vi "UI.vi"(8 "error in (no error)":errorcluster, 11 "Node Ptr":T1 format="%.0x") -> (0 "error out":errorcluster)   [LabVIEW 2017, in "Modules.lvlib" / "9210.lvclass"]
uses:
  9210.lvclass
  <vilib>/NI Veristand/Custom Device API/Custom Device Item Ref.ctl
  RSI Module/SubPanel Command.ctl
  C:/Users/nitest/Documents/NI/niveristand-scan-engine-module-libraries/Source/RSI Module/RSI Module.lvclass
  9210.lvclass/9210.ctl
  RSI Module/RSI Module.lvclass
  <vilib>/NI Veristand/Custom Device API/Custom Device API.lvlib
panel:
  in  "Units":u8(ring) caption="Measurement Units" items=["Raw Volts", "Degrees Kelvin", "Degrees Celsius", "Degrees Fahrenheit", "Degrees Rankine"]
  in  "Type":u8(ring) caption="Thermocouple Type" items=["J", "K", "T", "E", "R", "S", "N", "B"]
  in  "Channels":i32[](listbox)=[0]
  in  "SubPanel Event":refnum<user-event>
  in  "Header":cluster{"Section Name":string}={"Section Name"="NI 9210 Settings"}
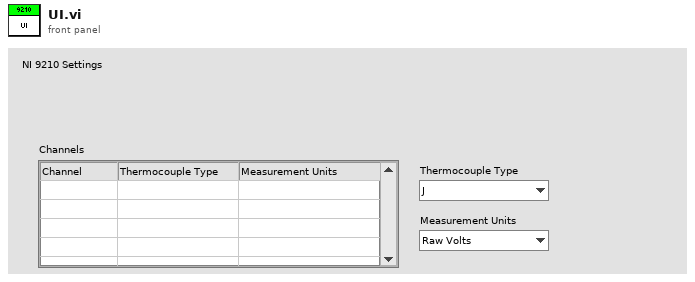
[diagram p1: front panel]
types:
  T1 = typedef "Custom Device API.lvlib/Custom Device Item Ref.ctl" = u64
  T2 = typedef "Modules.lvlib/RSI Module.lvclass/Module Models.ctl" = enum16{"Empty", "NI 9201", "NI 9203", "NI 9205", "NI 9206", "NI 9207", "NI 9208", "NI 9209", "NI 9210", "NI 9211", "NI 9212", "NI 9213", "NI 9214", "NI 9215", "NI 9216", "NI 9217", "NI 9219", "NI 9220", "NI 9221", "NI 9222", "NI 9223", "NI 9224", "NI 9225", "NI 9226", "NI 9227", "NI 9228", "NI 9229", "NI 9233", "NI 9234", "NI 9235", "NI 9236", "NI 9237", "NI 9239", "NI 9242", "NI 9244", "NI 9253", "NI 9263", "NI 9264", "NI 9265", "NI 9266", "NI 9269", "NI 9344", "NI 9350", "NI 9375", "NI 9401", "NI 9402", "NI 9403", "NI 9411", "NI 9421", "NI 9422", "NI 9423", "NI 9425", "NI 9426", "NI 9435", "NI 9436", "NI 9437", "NI 9472", "NI 9474", "NI 9475", "NI 9476", "NI 9477", "NI 9478", "NI 9481", "NI 9482", "NI 9485"}
  T3 = typedef "Modules.lvlib/RSI Module.lvclass/SubPanel Command.ctl" = enum16{"Stop"}
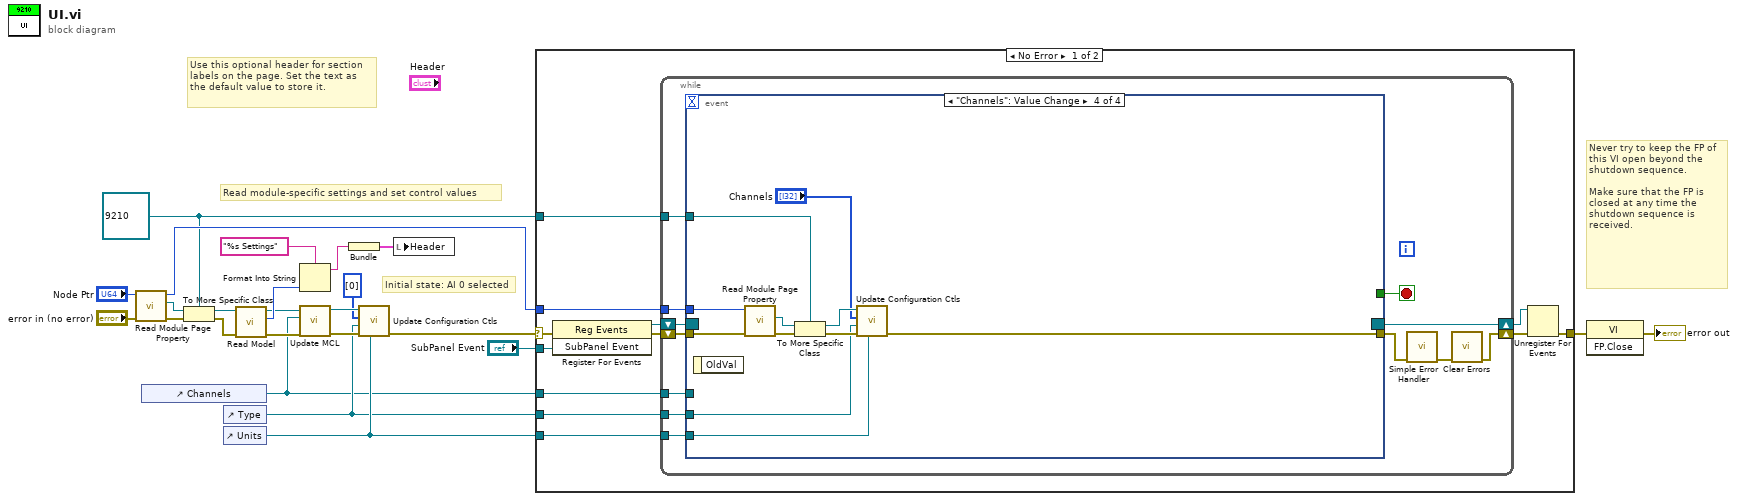
[diagram p0: block diagram]
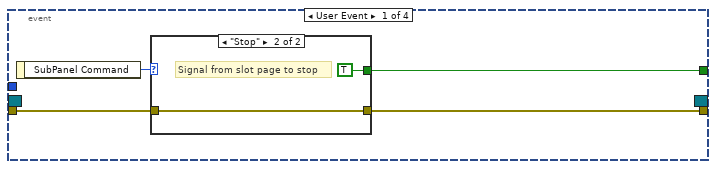
[diagram p2: hidden frame]
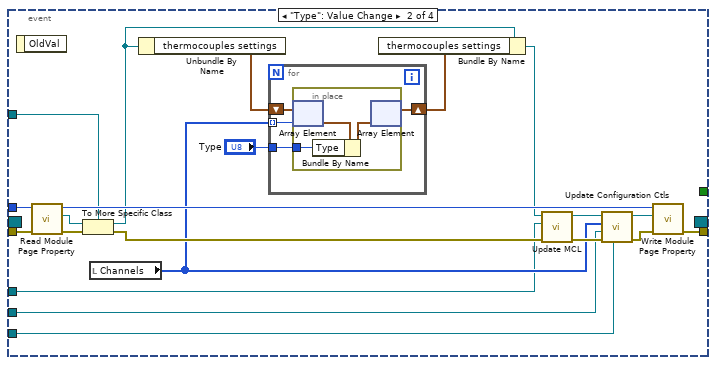
[diagram p4: hidden frame]
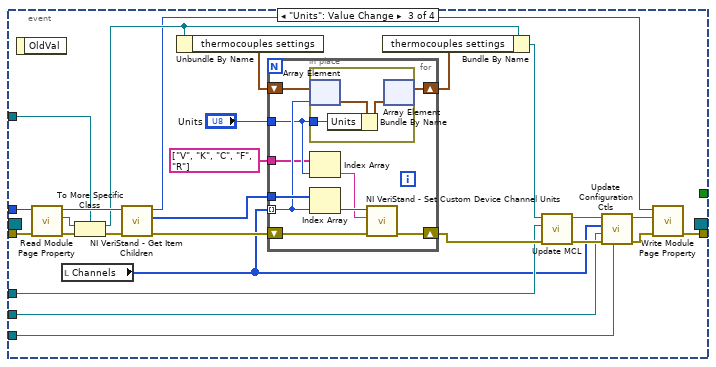
[diagram p5: hidden frame]
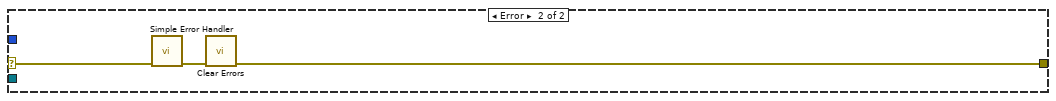
[diagram p6: hidden frame]
diagram:
  w1 = refnum<class "9210.lvclass"> refnum ("9205 in")
  # "Never try to keep the FP of this VI open beyond the shutdown sequence.\n\nMake sure that the FP is closed at any time the shutdown sequence is received."
  # "Initial state: AI 0 selected"
  # "Read module-specific settings and set control values"
  # "Use this optional header for section labels on the page. Set the text as the default value to store it."
  n1 = call "Read Module Page Property.vi"("error in (no error)"="error in (no error)", "Node Ptr In"="Node Ptr") -> ("error out"=w18:errorcluster, "RSI Module"=w17:refnum<class "RSI Module.lvclass">, "Node Ptr Out"=w21:T1)  [unwired: 7 in]
  n2 = control-ref of="Channels"() -> (w2:refnum<vi>)
  n3 = To More Specific Class(target class=w1, reference=w17, error in=w18) -> (specific class reference=w6:refnum<class "9210.lvclass">, error out=w7:errorcluster)
  n4 = control-ref of="Type"() -> (w3:refnum<vi>)
  n5 = control-ref of="Units"() -> (w4:refnum<vi>)
  n6 = call "Read Model.vi"("error in (no error)"=w7, "RSI Module in"=w6) -> ("error out"=w12:errorcluster, "Model"=w15:T2, "RSI Module out"=w11:refnum<class "9210.lvclass">)  [unwired: 7 in]
  n7 = Format Into String(format string="%s Settings", w15) -> (resulting string=w13:string)  [unwired: 2 in, 1 out]
  n8 = call "Update MCL.vi"("error in"=w12, "ListBox Refnum"=w2, "9210 in"=w11) -> ("error out"=w10:errorcluster, "9210 out"=w9:refnum<class "9210.lvclass">)  [unwired: 7 in]
  n9 = Bundle(w13) -> (w16:cluster{string})  [unwired: 1 in]
  n10 = call "Update Configuration Ctls.vi"("Units"=w4, "error in"=w10, "Type"=w3, "selected channels"=i32[] [0] ("Selected Channels"), "9210 in"=w9) -> ("error out"=w5:errorcluster)  [unwired: 5 in, 1 out]
  n11 = local write "Header"(w16) -> ()
  n12 = case shown="No Error" w5 {
    selector: w5 -> [w30 w136]
    tunnel: [w34 w134] -> w24
    tunnel: w21 -> [w31 _]
    tunnel: "SubPanel Event" -> [w29 _]
    tunnel: w4 -> [w28 _]
    tunnel: w3 -> [w27 _]
    tunnel: w2 -> [w26 _]
    tunnel: w1 -> [w25 _]
    frame No Error {
      n13 = register-events(error in=w30, w29) -> (reference out=w32:refnum<event-registration>, error out=w33:errorcluster)  [unwired: 1 in]
      n14 = while {
        tunnel: w31 -> [w44]
        shift-right: [w41] -> w35
        shift-left: w33 -> [w47]
        shift-right: [w48] -> w36
        shift-left: w32 -> [w46]
        tunnel: w25 -> [w40]
        tunnel: w28 -> [w39]
        tunnel: w27 -> [w38]
        tunnel: w26 -> [w37]
        stop <- w45 stop-if-true
        n15 = event shown="[3] \"Channels\": Value Change" {
          selector: w46 -> [_ _ _ _]
          dyn-events: [_ _ _ _] -> w48
          timeout: _ -> [_ _ _ _]
          tunnel: w47 -> [w51 w72 w106 w131]
          tunnel: [w50 _ _ _] -> w45
          tunnel: [w49 w71 w105 w127] -> w43
          tunnel: w44 -> [_ w73 w107 w130]
          tunnel: w40 -> [_ w65 w93 w123]
          tunnel: w39 -> [_ w63 w89 w124]
          tunnel: w38 -> [_ w64 w88 w125]
          tunnel: w37 -> [_ w56 w87 _]
          event User Event {
            n16 = event-data() -> ("SubPanel Command"=w52:T3)  [unwired: 1 out]
            n17 = case shown="\"Stop\"" w52 {
              tunnel: w51 -> [w53 w54]
              tunnel: [w53 w54] -> w49
              tunnel: [_ TRUE] -> w50
              frame Default {
              }
              frame "Stop" {
                # "Signal from slot page to stop"
              }
            }
          }
          event "Type": Value Change {
            n18 = event-data() -> ()  [unwired: 2 out]
            n19 = call "Read Module Page Property.vi"("error in (no error)"=w72, "Node Ptr In"=w73) -> ("error out"=w75:errorcluster, "RSI Module"=w76:refnum<class "RSI Module.lvclass">, "Node Ptr Out"=w74:T1)  [unwired: 7 in]
            n20 = To More Specific Class(target class=w65, reference=w76, error in=w75) -> (specific class reference=w60:refnum<class "9210.lvclass">, error out=w70:errorcluster)
            n21 = local read "Channels"() -> (w57:i32[])
            n22 = Unbundle By Name(w60) -> ("thermocouples settings"=w62:cluster{"Units":u8, "Type":u8}[])
            n23 = for {
              tunnel: w57 -> [w79] mode=indexing
              shift-right: [w77] -> w61
              shift-left: w62 -> [w80]
              tunnel: "Type" -> [w78]
              n24 = in-place {
                in-place-border: w78 -> [w82]
                n25 = in-place-array #1(w80, w79) -> (w83:cluster{"Units":u8, "Type":u8})
                n26 = Bundle By Name(cluster=w83, "Type"=w82) -> (w81:cluster{"Units":u8, "Type":u8})
                n27 = in-place-array #1(w81) -> (w77:cluster{"Units":u8, "Type":u8}[])  [unwired: 1 out]
              }
            }
            n28 = Bundle By Name(cluster=w60, "thermocouples settings"=w61) -> (w59:refnum<class "9210.lvclass">)
            n29 = call "Update MCL.vi"("error in"=w70, "ListBox Refnum"=w56, "9210 in"=w59) -> ("error out"=w69:errorcluster, "9210 out"=w67:refnum<class "9210.lvclass">)  [unwired: 7 in]
            n30 = call "Update Configuration Ctls.vi"("Units"=w63, "error in"=w69, "Type"=w64, "selected channels"=w57, "9210 in"=w67) -> ("error out"=w68:errorcluster, "9210 out"=w66:refnum<class "9210.lvclass">)  [unwired: 5 in]
            n31 = call "Write Module Page Property.vi"("error in (no error)"=w68, "RSI Module"=w66, "Node Ptr In"=w74) -> ("error out"=w71:errorcluster)  [unwired: 6 in, 2 out]
          }
          event "Units": Value Change {
            n32 = event-data() -> ()  [unwired: 2 out]
            n33 = call "Read Module Page Property.vi"("error in (no error)"=w106, "Node Ptr In"=w107) -> ("error out"=w108:errorcluster, "RSI Module"=w109:refnum<class "RSI Module.lvclass">, "Node Ptr Out"=w98:T1)  [unwired: 7 in]
            n34 = local read "Channels"() -> (w86:i32[])
            n35 = To More Specific Class(target class=w93, reference=w109, error in=w108) -> (specific class reference=w85:refnum<class "9210.lvclass">, error out=w99:errorcluster)
            n36 = call <vilib>:"NI VeriStand - Get Item Children.vi"("error in (no error)"=w99, "Item Ref in"=w98) -> ("error out"=w96:errorcluster, "Child Refs"=w97:T1[], "Item Ref out"=w84:T1)  [unwired: 6 in, 1 out]
            n37 = Unbundle By Name(w85) -> ("thermocouples settings"=w92:cluster{"Units":u8, "Type":u8}[])
            n38 = for {
              tunnel: w86 -> [w113] mode=indexing
              shift-right: [w111] -> w91
              shift-left: w92 -> [w114]
              tunnel: "Units" -> [w112]
              shift-right: [w116] -> w95
              shift-left: w96 -> [w117]
              tunnel: w97 -> [w119]
              tunnel: string[] ["V", "K", "C", "F", "R"] -> [w110]
              n39 = in-place {
                in-place-border: w112 -> [w121]
                n40 = in-place-array #2(w114, w113) -> (w122:cluster{"Units":u8, "Type":u8})
                n41 = Bundle By Name(cluster=w122, "Units"=w121) -> (w120:cluster{"Units":u8, "Type":u8})
                n42 = in-place-array #2(w120) -> (w111:cluster{"Units":u8, "Type":u8}[])  [unwired: 1 out]
              }
              n43 = Index Array(array=w110, index=w112) -> (element=w115:string)
              n44 = Index Array(array=w119, index=w113) -> (element=w118:T1)
              n45 = call <vilib>:"NI VeriStand - Set Custom Device Channel Units.vi"("error in (no error)"=w117, "Units"=w115, "Channel Ref in"=w118) -> ("error out"=w116:errorcluster)  [unwired: 7 in, 1 out]
            }
            n46 = Bundle By Name(cluster=w85, "thermocouples settings"=w91) -> (w90:refnum<class "9210.lvclass">)
            n47 = call "Update MCL.vi"("error in"=w95, "ListBox Refnum"=w87, "9210 in"=w90) -> ("error out"=w104:errorcluster, "9210 out"=w102:refnum<class "9210.lvclass">)  [unwired: 7 in]
            n48 = call "Update Configuration Ctls.vi"("Units"=w89, "error in"=w104, "Type"=w88, "selected channels"=w86, "9210 in"=w102) -> ("error out"=w103:errorcluster, "9210 out"=w100:refnum<class "9210.lvclass">)  [unwired: 5 in]
            n49 = call "Write Module Page Property.vi"("error in (no error)"=w103, "RSI Module"=w100, "Node Ptr In"=w84) -> ("error out"=w105:errorcluster)  [unwired: 6 in, 2 out]
          }
          event "Channels": Value Change {
            n50 = event-data() -> ()  [unwired: 2 out]
            n51 = call "Read Module Page Property.vi"("error in (no error)"=w131, "Node Ptr In"=w130) -> ("error out"=w132:errorcluster, "RSI Module"=w133:refnum<class "RSI Module.lvclass">)  [unwired: 7 in, 1 out]
            n52 = To More Specific Class(target class=w123, reference=w133, error in=w132) -> (specific class reference=w128:refnum<class "9210.lvclass">, error out=w129:errorcluster)
            n53 = call "Update Configuration Ctls.vi"("Units"=w124, "error in"=w129, "Type"=w125, "selected channels"="Channels", "9210 in"=w128) -> ("error out"=w127:errorcluster)  [unwired: 5 in, 1 out]
          }
        }
        n54 = call <vilib>:"Simple Error Handler.vi"("error in (no error)"=w43) -> ("error out"=w42:errorcluster)  [unwired: 1 in, 7 out]
        n55 = call <vilib>:"Clear Errors.vi"("error in (no error)"=w42) -> ("error out"=w41:errorcluster)  [unwired: 1 in, 5 out]
      }
      n56 = Unregister For Events(event registration refnum=w36, error in=w35) -> (error out=w34:errorcluster)
    }
    frame Error {
      n57 = call <vilib>:"Simple Error Handler.vi"("error in (no error)"=w136) -> ("error out"=w135:errorcluster)  [unwired: 1 in, 7 out]
      n58 = call <vilib>:"Clear Errors.vi"("error in (no error)"=w135) -> ("error out"=w134:errorcluster)  [unwired: 1 in, 5 out]
    }
  }
  n59 = invoke class="VI" method="FP.Close"(error in=w24) -> (error out=→"error out":errorcluster)  [unwired: 2 in, 2 out]
